vi "Ch_data_pattern_16_save (SubVI).vi"(7 "error in":errorcluster, 10 "R1-8 Cluster":T1, 11 "P S1":dbl, 12 "T1-8 Cluster":T2, 13 "P S2":dbl, 14 "R9-16":T1, 15 "Activate!":bool, 16 "T9-16":T2, 17 "file":refnum<file>) -> (27 "error out":errorcluster)   [LabVIEW 2013]
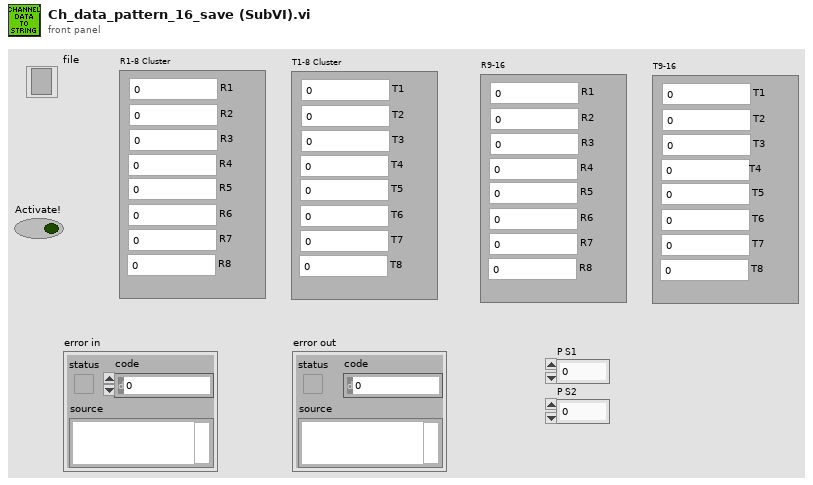
[diagram p1: front panel]
types:
  T1 = cluster{"R1":dbl, "R2":dbl, "R3":dbl, "R4":dbl, "R5":dbl, "R6":dbl, "R7":dbl, "R8":dbl}
  T2 = cluster{"T1":dbl, "T2":dbl, "T3":dbl, "T4":dbl, "T5":dbl, "T6":dbl, "T7":dbl, "T8":dbl}
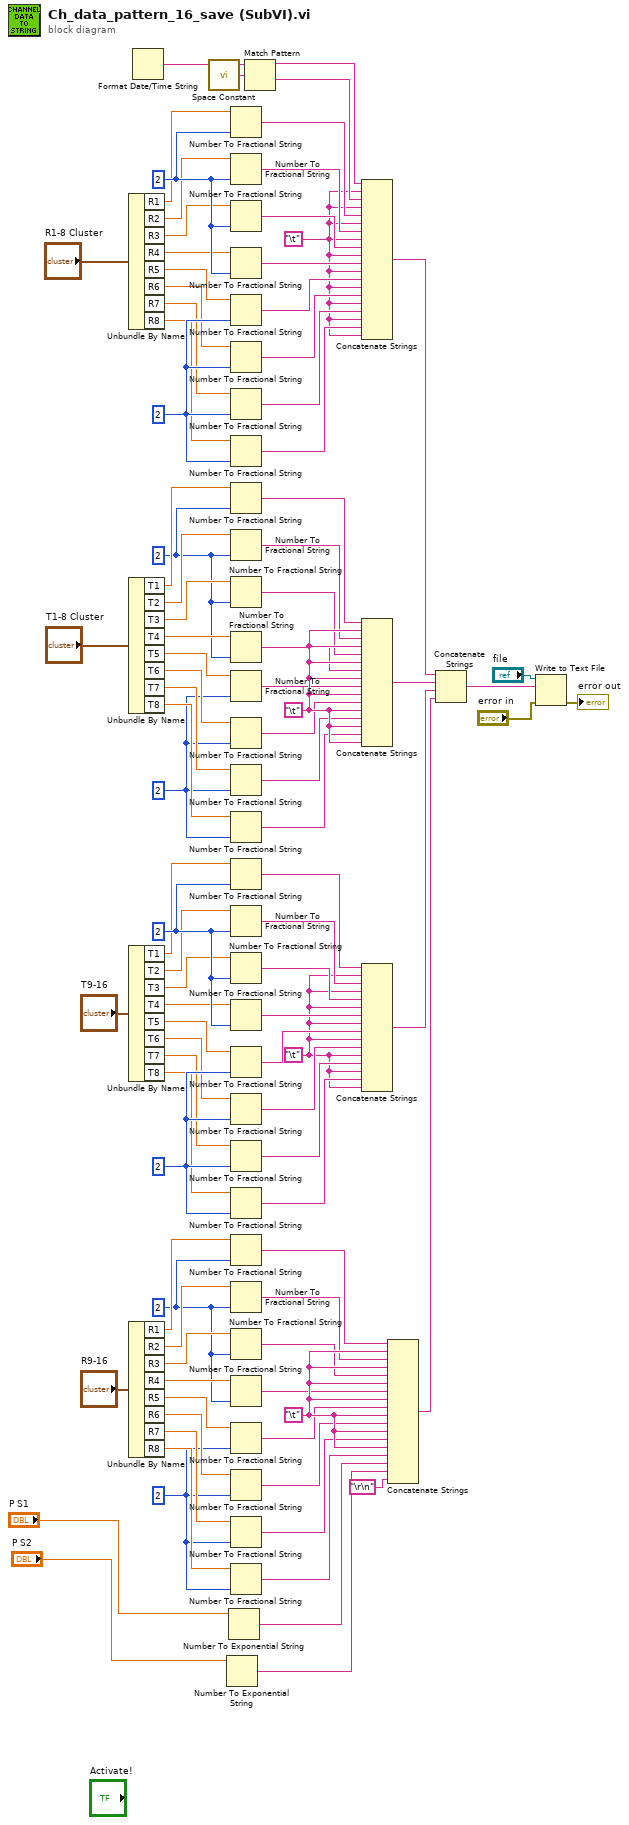
[diagram p0: block diagram]
diagram:
  w40 = i16 2 ("precision (6)")
  w44 = i16 2 ("precision (6)")
  w27 = "\t"
  w13 = i16 2 ("precision (6)")
  w8 = i16 2 ("precision (6)")
  w26 = "\t"
  w57 = i16 2 ("precision (6)")
  w53 = i16 2 ("precision (6)")
  w70 = "\t"
  w86 = i16 2 ("precision (6)")
  w96 = i16 2 ("precision (6)")
  w73 = "\t"
  n1 = Unbundle By Name("R1-8 Cluster") -> ("R1"=w81:dbl, "R2"=w80:dbl, "R3"=w79:dbl, "R4"=w78:dbl, "R5"=w77:dbl, "R6"=w76:dbl, "R7"=w75:dbl, "R8"=w74:dbl)
  n2 = Unbundle By Name("T1-8 Cluster") -> ("T1"=w62:dbl, "T2"=w63:dbl, "T3"=w64:dbl, "T4"=w65:dbl, "T5"=w66:dbl, "T6"=w67:dbl, "T7"=w68:dbl, "T8"=w69:dbl)
  n3 = Unbundle By Name("T9-16") -> ("T1"=w35:dbl, "T2"=w34:dbl, "T3"=w33:dbl, "T4"=w32:dbl, "T5"=w31:dbl, "T6"=w30:dbl, "T7"=w29:dbl, "T8"=w28:dbl)
  n4 = Unbundle By Name("R9-16") -> ("R1"=w18:dbl, "R2"=w19:dbl, "R3"=w20:dbl, "R4"=w21:dbl, "R5"=w22:dbl, "R6"=w23:dbl, "R7"=w24:dbl, "R8"=w25:dbl)
  n5 = Format Date/Time String() -> (date/time string=w88:string)  [unwired: 3 out]
  n6 = call <vilib>:"Space Constant.vi"() -> ("String"=w89:string)
  n7 = Number To Exponential String(number="P S2") -> (E-format string=w1:string)  [unwired: 3 in]
  n8 = Number To Exponential String(number="P S1") -> (E-format string=w3:string)  [unwired: 3 in]
  n9 = Number To Fractional String(number=w81, precision (6)=w96) -> (F-format string=w92:string)  [unwired: 2 out]
  n10 = Number To Fractional String(number=w80, precision (6)=w96) -> (F-format string=w93:string)  [unwired: 2 out]
  n11 = Number To Fractional String(number=w79, precision (6)=w96) -> (F-format string=w94:string)  [unwired: 2 out]
  n12 = Number To Fractional String(number=w78, precision (6)=w96) -> (F-format string=w95:string)  [unwired: 2 out]
  n13 = Number To Fractional String(number=w77, precision (6)=w86) -> (F-format string=w85:string)  [unwired: 2 out]
  n14 = Number To Fractional String(number=w76, precision (6)=w86) -> (F-format string=w84:string)  [unwired: 2 out]
  n15 = Number To Fractional String(number=w75, precision (6)=w86) -> (F-format string=w83:string)  [unwired: 2 out]
  n16 = Number To Fractional String(number=w74, precision (6)=w86) -> (F-format string=w82:string)  [unwired: 2 out]
  n17 = Number To Fractional String(number=w62, precision (6)=w53) -> (F-format string=w56:string)  [unwired: 2 out]
  n18 = Number To Fractional String(number=w63, precision (6)=w53) -> (F-format string=w50:string)  [unwired: 2 out]
  n19 = Number To Fractional String(number=w64, precision (6)=w53) -> (F-format string=w55:string)  [unwired: 2 out]
  n20 = Number To Fractional String(number=w65, precision (6)=w53) -> (F-format string=w54:string)  [unwired: 2 out]
  n21 = Number To Fractional String(number=w66, precision (6)=w57) -> (F-format string=w58:string)  [unwired: 2 out]
  n22 = Number To Fractional String(number=w67, precision (6)=w57) -> (F-format string=w59:string)  [unwired: 2 out]
  n23 = Number To Fractional String(number=w68, precision (6)=w57) -> (F-format string=w60:string)  [unwired: 2 out]
  n24 = Number To Fractional String(number=w69, precision (6)=w57) -> (F-format string=w61:string)  [unwired: 2 out]
  n25 = Number To Fractional String(number=w35, precision (6)=w44) -> (F-format string=w41:string)  [unwired: 2 out]
  n26 = Number To Fractional String(number=w34, precision (6)=w44) -> (F-format string=w45:string)  [unwired: 2 out]
  n27 = Number To Fractional String(number=w33, precision (6)=w44) -> (F-format string=w42:string)  [unwired: 2 out]
  n28 = Number To Fractional String(number=w32, precision (6)=w44) -> (F-format string=w43:string)  [unwired: 2 out]
  n29 = Number To Fractional String(number=w31, precision (6)=w40) -> (F-format string=w39:string)  [unwired: 2 out]
  n30 = Number To Fractional String(number=w30, precision (6)=w40) -> (F-format string=w38:string)  [unwired: 2 out]
  n31 = Number To Fractional String(number=w29, precision (6)=w40) -> (F-format string=w37:string)  [unwired: 2 out]
  n32 = Number To Fractional String(number=w28, precision (6)=w40) -> (F-format string=w36:string)  [unwired: 2 out]
  n33 = Number To Fractional String(number=w18, precision (6)=w8) -> (F-format string=w12:string)  [unwired: 2 out]
  n34 = Number To Fractional String(number=w19, precision (6)=w8) -> (F-format string=w11:string)  [unwired: 2 out]
  n35 = Number To Fractional String(number=w20, precision (6)=w8) -> (F-format string=w10:string)  [unwired: 2 out]
  n36 = Number To Fractional String(number=w21, precision (6)=w8) -> (F-format string=w9:string)  [unwired: 2 out]
  n37 = Number To Fractional String(number=w22, precision (6)=w13) -> (F-format string=w14:string)  [unwired: 2 out]
  n38 = Number To Fractional String(number=w23, precision (6)=w13) -> (F-format string=w15:string)  [unwired: 2 out]
  n39 = Number To Fractional String(number=w24, precision (6)=w13) -> (F-format string=w16:string)  [unwired: 2 out]
  n40 = Number To Fractional String(number=w25, precision (6)=w13) -> (F-format string=w17:string)  [unwired: 2 out]
  n41 = Match Pattern(string=w88, regular expression=w89) -> (before substring=w90:string, after substring=w91:string)  [unwired: 3 out]
  n42 = Concatenate Strings(w90, w73, w91, w73, w92, w73, w93, w73, w94, w73, w95, w73, w85, w73, w84, w73, w83, w73, w82, w73) -> (w72:string)
  n43 = Concatenate Strings(w56, w70, w50, w70, w55, w70, w54, w70, w58, w70, w59, w70, w60, w70, w61, w70) -> (w52:string)
  n44 = Concatenate Strings(w41, w27, w45, w27, w42, w27, w43, w27, w39, w27, w38, w27, w37, w27, w36, w27) -> (w7:string)
  n45 = Concatenate Strings(w12, w26, w11, w26, w10, w26, w9, w26, w14, w26, w15, w26, w16, w26, w17, w3, w1, "\r\n") -> (w6:string)
  n46 = Concatenate Strings(w72, w52, w7, w6) -> (w71:string)
  n47 = Write to Text File(file (use dialog)="file", text=w71, error in="error in") -> (error out=→"error out":errorcluster)  [unwired: 3 out]
